vi "h5timestamp.vi"   [LabVIEW 2011]
uses:
  <instrlib>/niHWS/nihws.llb/niHWS Read Analog WDT.vi
types:
  T1 = typedef "LVDateTimeRec.ctl" = cluster{"fractional second":dbl, "second":i32, "minute":i32, "hour":i32, "day of month":i32, "month":i32, "year":i32, "day of week":i32, "day of year":i32, "DST":i32}
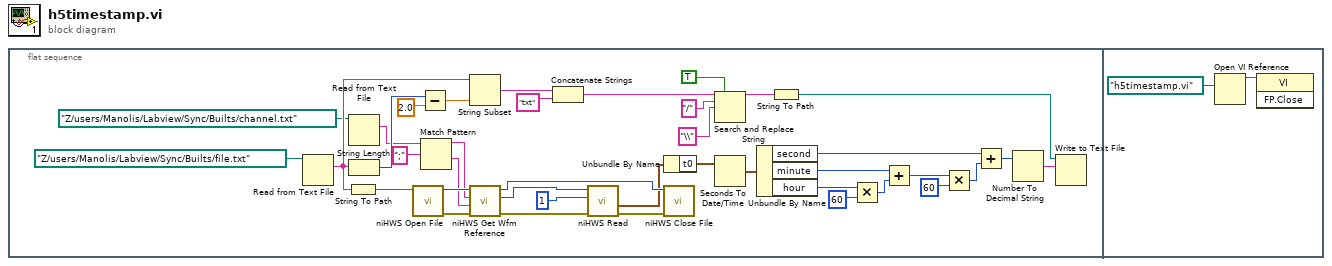
[diagram p0: block diagram]
diagram:
  n1 = flat-sequence {
    frame #0 {
      n2 = Read from Text File(file (use dialog)=path "Z:/users/Manolis/Labview/Sync/Builts/file.txt") -> (text=w16:string)  [unwired: 3 in, 3 out]
      n3 = String To Path(string=w16) -> (path=w20:path)
      n4 = Read from Text File(file (use dialog)=path "Z:/users/Manolis/Labview/Sync/Builts/channel.txt") -> (text=w4:string)  [unwired: 3 in, 3 out]
      n5 = String Length(string=w16) -> (length=w14:i32)
      n6 = call <instrlib>:"niHWS Open File.vi"("file path"=w20) -> ("error out"=w39:errorcluster, "file handle"=w35:u32)  [unwired: 9 in]
      n7 = Subtract(x=w14, y=2.0) -> (x-y=w13:dbl)
      n8 = Match Pattern(string=w4, regular expression=";") -> (before substring=w2:string, after substring=w1:string)  [unwired: 1 in, 2 out]
      n9 = String Subset(string=w16, length (rest)=w13) -> (substring=w12:string)  [unwired: 1 in]
      n10 = call <instrlib>:"niHWS Get Wfm Reference.vi"("error in (no error)"=w39, "waveform name (empty)"=w1, "group name (empty)"=w2, "file handle in"=w35) -> ("error out"=w34:errorcluster, "waveform reference"=w38:u32, "file handle out"=w37:u32)  [unwired: 5 in]
      n11 = Concatenate Strings(w12, "txt" ("string")) -> (w10:string)
      n12 = call-poly <instrlib>:"niHWS Read.vi"("error in (no error)"=w34, "num samples to read (-1:all)"=1, "waveform reference in"=w38) -> ("error out"=w33:errorcluster, "analog waveform"=w36:waveform(dbl))  [unwired: 5 in, 2 out]
      n13 = Unbundle By Name(w36) -> ("t0"=w31:timestamp)
      n14 = call <instrlib>:"niHWS Close File.vi"("error in (no error)"=w33, "file handle"=w37) -> ()  [unwired: 9 in, 1 out]
      n15 = Search and Replace String(replace all?=TRUE ("replace all? (F)"), input string=w10, search string="/", replace string="\\" ("replace string (\"\")")) -> (result string=w9:string)  [unwired: 4 in, 3 out]
      n16 = Seconds To Date/Time(time stamp (now)=w31) -> (date time rec=w30:T1)  [unwired: 1 in]
      n17 = Unbundle By Name(w30) -> ("second"=w24:i32, "minute"=w29:i32, "hour"=w27:i32)
      n18 = String To Path(string=w9) -> (path=w17:path)
      n19 = Multiply(x=w27, y=60) -> (x*y=w28:i32)
      n20 = Add(x=w29, y=w28) -> (x+y=w23:i32)
      n21 = Multiply(x=w23, y=60) -> (x*y=w22:i32)
      n22 = Add(x=w24, y=w22) -> (x+y=w19:i32)
      n23 = Number To Decimal String(number=w19) -> (decimal integer string=w18:string)  [unwired: 1 in]
      n24 = Write to Text File(file (use dialog)=w17, text=w18) -> ()  [unwired: 2 in, 3 out]
    }
    frame #1 {
      n25 = Open VI Reference(vi path=path "h5timestamp.vi") -> (vi reference=w40:refnum<vi>)  [unwired: 5 in, 1 out]
      n26 = invoke class="VI" method="FP.Close"(reference=w40) -> ()  [unwired: 2 in, 3 out]
    }
  }
